vi "RSZVB Select Stability Factors.vi"(5 "DUT Out (2)":i32=2, 6 "Stability Factor (0: K)":i32(ring) items=["K", "u1", "u2"], 7 "DUT In (1)":i32=1, 8 "error in (no error)":errorcluster {"code" format="%.0x"}, 9 "Trace Name (Trc1)":string="Trc1", 10 "Channel (1)":i32=1, 11 "VISA session":refnum<visa-resource-name>) -> (0 "error out":errorcluster {"code" format="%.0x"}, 3 "dup VISA session":refnum<visa-resource-name>)   [LabVIEW 2011]
doc: "This VI select one of the three two port stability factors K, u1 or u2.\n\nStability factors are calculated as VIs of the frequency or another stimulus parameter. They provide criteria for linear stability of two-ports such as amplifiers. A linear circuit is said to be unconditionally stable if no combination of passive source or load can cause the circuit to oscillate.\n\nAssigns a measurement parameter to an existing trace or creates a trace and assigns a channel number, a name and a measurement parameter to it. The trace is not displayed.\n\nStability factors can be calculated for unbalanced ports only. If a balanced port configuration is selected, the analyzer generates an error message.\n\nRemote-control command(s):\nCALCulate<Ch>:PARameter:SDEFine '<string>', 'KFAC21' | 'MUF121' | 'MUF221' | ...\nCALCulate<Ch>:PARameter:MEASure '<string>', 'KFAC21' | 'MUF121' | 'MUF221' | ..."
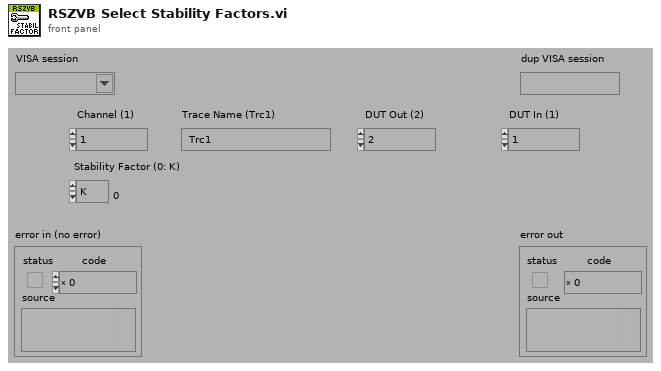
[diagram p1: front panel]
types:
  T1 = cluster{"Error Checking (T: On)":bool, "Installed Options":string[], "Data Valid?":bool, "Ports":i32, "Model":string[], "Option Checking (T: On)":bool}
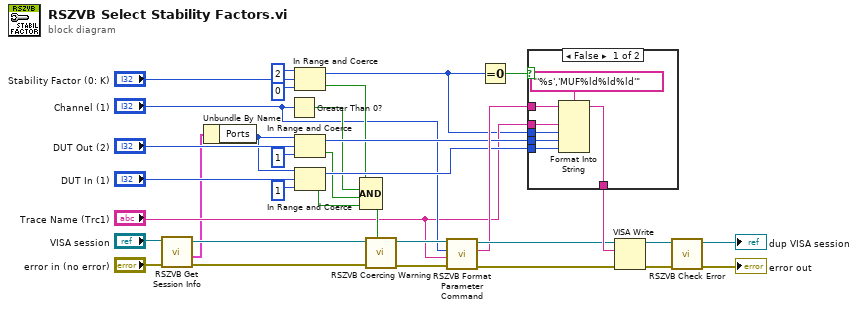
[diagram p0: block diagram]
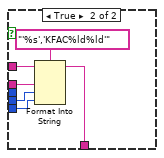
[diagram p2: hidden frame]
diagram:
  n1 = call "RSZVB Get Session Info.vi"("error in (no error)"="error in (no error)", "VISA session"="VISA session") -> ("error out"=w4:errorcluster, "Session Info"=w2:T1, "dup VISA session"=w3:refnum<visa-resource-name>)  [unwired: 7 in]
  n2 = Unbundle By Name(w2) -> ("Ports"=w1:i32)
  n3 = Greater Than 0?(x="Channel (1)") -> (x > 0?=w19:bool)
  n4 = In Range and Coerce(upper limit=2, x="Stability Factor (0: K)", lower limit=0) -> (coerced(x)=w7:i32, In Range?=w20:bool)
  n5 = In Range and Coerce(upper limit=w1, x="DUT Out (2)", lower limit=1) -> (coerced(x)=w22:i32, In Range?=w18:bool)
  n6 = In Range and Coerce(upper limit=w1, x="DUT In (1)", lower limit=1) -> (coerced(x)=w21:i32, In Range?=w17:bool)
  n7 = Compound Arithmetic op=AND(w20, w19, w18, w17) -> (w31:bool)
  n8 = call "RSZVB Coercing Warning.vi"("In Range?"=w31, "error in (no error)"=w4, "VISA session"=w3) -> ("error out"=w28:errorcluster, "dup VISA session"=w27:refnum<visa-resource-name>)  [unwired: 7 in]
  n9 = call "RSZVB Format Parameter Command.vi"("error in (no error)"=w28, "Trace Name (Trc1)"="Trace Name (Trc1)", "Channel (1)"="Channel (1)", "VISA session"=w27) -> ("error out"=w29:errorcluster, "Buffer"=w25:string, "dup VISA session"=w26:refnum<visa-resource-name>)  [unwired: 5 in]
  n10 = Equal To 0?(x=w7) -> (x = 0?=w8:bool)
  n11 = case shown="False" w8 {
    tunnel: [w38 w46] -> w30
    tunnel: w25 -> [w39 w45]
    tunnel: w22 -> [w36 w44]
    tunnel: w21 -> [w35 w43]
    tunnel: "Trace Name (Trc1)" -> [w40 w42]
    tunnel: w7 -> [w37 _]
    frame False {
      n12 = Format Into String(format string="'%s','MUF%ld%ld%ld'", initial string=w39, w40, w37, w36, w35) -> (resulting string=w38:string)  [unwired: 1 in, 1 out]
    }
    frame True {
      n13 = Format Into String(format string="'%s','KFAC%ld%ld'", initial string=w45, w42, w44, w43) -> (resulting string=w46:string)  [unwired: 1 in, 1 out]
    }
  }
  n14 = VISA Write(VISA resource name=w26, write buffer=w30, error in (no error)=w29) -> (VISA resource name out=w32:refnum<visa-resource-name>, error out=w33:errorcluster)  [unwired: 1 out]
  n15 = call "RSZVB Check Error.vi"("error in (no error)"=w33, "VISA session"=w32) -> ("error out"=→"error out":errorcluster, "dup VISA session"=→"dup VISA session":refnum<visa-resource-name>)  [unwired: 8 in]
